vi "TestPlunger.vi"() -> ()   [LabVIEW 2011]
panel:
  in  "toogle":bool=TRUE
  in  "output 1":T1(ring)
  in  "stop":bool
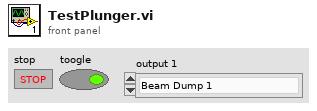
[diagram p1: front panel]
types:
  T1 = enum16{"Beam Dump 1", "Beam Dump 2", "Wedge", "Phosphor"}
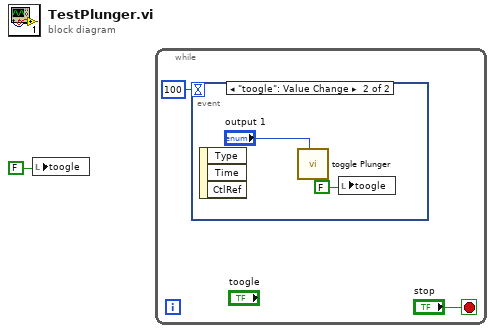
[diagram p0: block diagram]
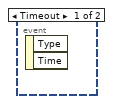
[diagram p2: hidden frame]
diagram:
  n1 = local write "toogle"(FALSE ("toogle")) -> ()
  n2 = while {
    stop <- "stop" stop-if-true
    n3 = event shown="[1] \"toogle\": Value Change" {
      selector: _ -> [_ _]
      dyn-events: _ -> [_ _]
      timeout: 100 -> [_ _]
      event Timeout {
        n4 = event-data() -> ()  [unwired: 1 in, 2 out]
      }
      event "toogle": Value Change {
        n5 = event-data() -> ()  [unwired: 1 in, 3 out]
        n6 = call "toggle Plunger.vi"("Plunger"="output 1") -> ()  [unwired: 10 in, 1 out]
        n7 = local write "toogle"(FALSE ("toogle")) -> ()
      }
    }
  }
